vi "Internal Operation.vi"(7 "Archt Map":variant, 8 "source/target":string, 9 "args":string, 10 "state":string, 11 "Numeric in":i32) -> (0 "error out":errorcluster, 3 "Numeric out":i32)   [LabVIEW 2020, in "CSMStand(Lite).lvlib"]
uses:
  CSMStand(Lite).lvlib
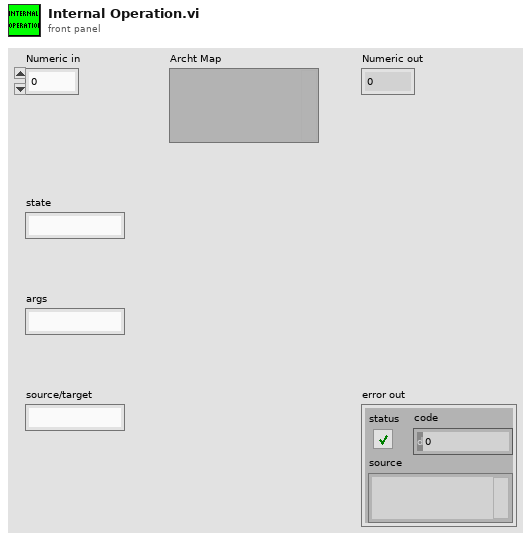
[diagram p1: front panel]
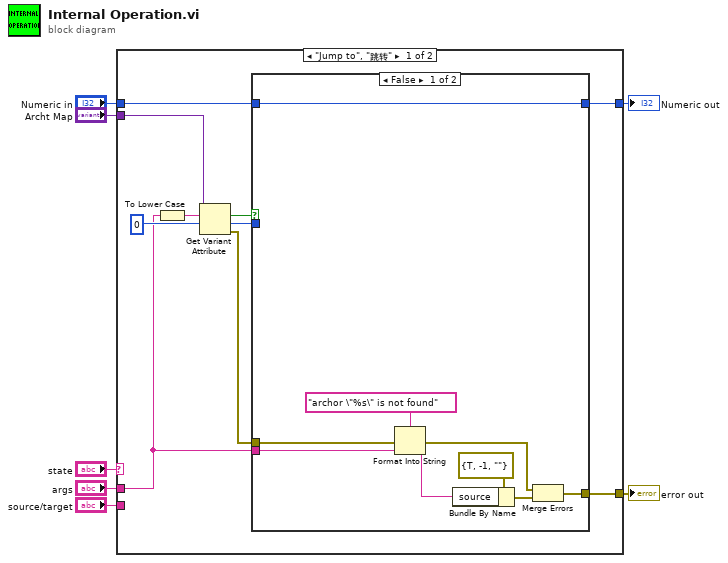
[diagram p0: block diagram]
diagram:
  n1 = case shown="\"Jump to\", \"跳转\"" "state" {
    tunnel: "args" -> [w11 _]
    tunnel: "source/target" -> [_ _]
    tunnel: [w14 w28] -> w4
    tunnel: "Numeric in" -> [w13 w28]
    tunnel: "Archt Map" -> [w17 _]
    tunnel: [w10 _] -> w7
    frame "Jump to", "跳转" {
      n2 = To Lower Case(string=w11) -> (all lower case string=w8:string)
      n3 = Get Variant Attribute(Variant=w17, name=w8, default value (empty Variant)=0) -> (found=w12:bool, value=w15:i32, error out=w9:errorcluster)  [unwired: 1 in, 1 out]
      n4 = case shown="False" w12 {
        tunnel: w15 -> [_ w27]
        tunnel: [w18 w27] -> w14
        tunnel: w13 -> [w18 _]
        tunnel: w11 -> [w24 _]
        tunnel: [w20 _] -> w10
        tunnel: w9 -> [w21 _]
        frame False {
          n5 = Format Into String(format string="archor \"%s\" is not found" ("source"), error in=w21, w24) -> (resulting string=w23:string, error out=w19:errorcluster)  [unwired: 1 in]
          n6 = Bundle By Name(cluster=errorcluster {"status"=TRUE, "code"=-1, "source"=""} ("error in (no error)"), "source"=w23) -> (w22:errorcluster)
          n7 = Merge Errors(w19, w22) -> (w20:errorcluster)
        }
        frame True {
        }
      }
    }
    frame Default {
    }
  }
  "error out" <- w7
  "Numeric out" <- w4
